vi "SPECAN_DPD_AMPM_ACP_TXP.vi"() -> ()   [LabVIEW 2016]
doc: "This example illustrates how to use the RFmx SpecAn and LTE personalities together with the RFSG drivers to perform ACP and EVM measurements with or without digital predistortion (DPD) of the waveform input to the DUT. \n\nDPD is a technique to optimize the operating point of power amplifiers and other non-linear RFIC devices. Power amplifiers are much more efficient if they operate near compression. However, compressing signal amplitudes can significantly deteriorate the amplified signal's quality both, in-band (e.g., EVM increases due to non-linear distortion of the signal's I/Q constellation) and out-of-band (e.g., ACP or SEM test fails due to spectral regrowth). With DPD, the original waveform is first pre-distorted in a way that matches the non-linear effects of the RFIC device before being fed through the device. The resulting output is a much cleaner amplified and/or filtered version of the original waveform. \n\nDifferent DPD models can be used to trade off performance with computational ease, with the Lookup-Table (LUT) model the simplest and the Generalized Memory Polynomial Model (GMP) the most complex. With a LUT, the DPD algorithm achieves gain and phase linearization on average. If you want to correct for memory effects - i.e., an output sample not only depends on the current input but also previous input samples; you will notice that a specific input power value translates into a range of gain and phase values - you would use one of the memory polynomial models. For these models, several parameters such as polynomial order and memory depth are available to fine-tune the model to the DUT behavior."
uses:
  <instrlib>/niRFSG/niRFSG.llb/niRFSG Exported Signal Destinations.ctl
  Source/SG/Typedefs/Instrument Configuration.ctl
  <instrlib>/niRFSG/niRFSG.llb/niRFSG Ref Clock Sources.ctl
  Source/Common/Local Oscillator Sharing Mode.ctl
  Source/SA/RFmxSpecAn/Typedefs/SpecAn AMPM Configuration.ctl
  Source/Common/Waveform.ctl
  Source/SA/RFmxSpecAn/Typedefs/SpecAn AMPM Results.ctl
  Source/Common/SA Common Configuration.ctl
  Source/SA/RFmxSpecAn/Typedefs/SpecAn ACP Configuration.ctl
  Source/SA/RFmxSpecAn/Typedefs/SpecAn ACP Component Carrier Configuration.ctl
  Source/SA/RFmxSpecAn/Typedefs/SpecAn ACP Offset Channel Configuration.ctl
  Source/SA/RFmxSpecAn/Typedefs/SpecAn ACP Offset Results.ctl
  Source/SA/RFmxSpecAn/Typedefs/SpecAn ACP Component Carrier Results.ctl
  Source/SA/RFmxSpecAn/Typedefs/SpecAn TxP Configuration.ctl
  Source/SA/RFmxSpecAn/Typedefs/SpecAn TxP Results.ctl
  Source/Methods/RFmxDPD/Typedefs/Common Configuration.ctl
  Source/Methods/RFmxDPD/Typedefs/Memory Polynomial Configuration.ctl
  Source/SA/RFmxInstr/Typedefs/Instrument Configuration.ctl
  Source/Methods/RFmxDPD/Typedefs/Pre DPD Crest Factor Reduction Configuration.ctl
  Source/Methods/RFmxDPD/Typedefs/Pre DPD Crest Factor Reduction Carrier Channel.ctl
  Source/Methods/RFmxDPD/Typedefs/Apply DPD Crest Factor Reduction Configuration.ctl
  Source/Common/SA Auto Level Configuration.ctl
  <vilib>/RFmx/SpecAn/mx/RFmxSpecAn.llb/RFmxSpecAn AMPM Fetch AM to AM Trace.vi
  <vilib>/RFmx/SpecAn/mx/RFmxSpecAn.llb/RFmxSpecAn AMPM Fetch AM to PM Trace.vi
  <vilib>/RFmx/SpecAn/mx/RFmxSpecAn.llb/RFmxSpecAn ACP Fetch Spectrum.vi
  <vilib>/RFmx/SpecAn/mx/RFmxSpecAn.llb/RFmxSpecAn TXP Fetch Power Trace.vi
  Source/SG/SG.lvlib
  Source/SA/RFmxSpecAn/RFmxSpecAn.lvlib
  Source/Methods/RFmxDPD/RFmxDPD.lvlib
  Source/SA/RFmxInstr/RFmxInstr.lvlib
  Source/Common/Common.lvlib
panel:
  in  "Display Tab Control":enum32{"AMPM Results", "ACP Results", "TxP"}(tab)
  out "AM to AM Plot":T1(graph)
  out "AM to PM Plot":T2(graph)
  out "AMPM Measurement Results":T3 {"AM to PM Residual (deg)" format="%.2f"; "AM to AM Residual (dB)" format="%.2f"; "Mean RMS EVM (%)" format="%.2f"; "1 dB Compression Point (dBm)" format="%.2f"; "Mean Linear Gain (dB)" format="%.2f"}
  out "Spectrum":cluster{"x0":dbl, "dx":dbl, "y":sgl[]}(graph) caption="DUT Output Spectrum"
  out "Offset Results":T4[](array[typedef])
  out "Component Carrier Results":T5[](array[typedef])
  out "Total Carrier Power (dBm or dBm/Hz)":dbl
  out "Power Trace":cluster{"x0":dbl, "dx":dbl, "y":sgl[]}(graph)
  out "TxP Results":T6 {"Minimum Power (dBm)" format="%.2f"; "Maximum Power (dBm)" format="%.2f"; "Peak to Average Ratio (dB)" format="%.2f"; "Average Mean Power (dBm)" format="%.2f"}
  in  "Measurement Settings Tab Control":T7(tab)
  in  "TxP Config":T8={"Measurement Interval (s)"=0.001, "RBW (Hz)"=20000000.0, "RBW Filter Type"=5, "RRC Alpha"=0.0, "Averaging Enabled"=0, "Averaging Count"=10, "Averaging Type"=0} {"Averaging Type" items=["RMS", "Log", "Scalar", "Max", "Min"]; "Averaging Enabled" items=["False", "True"]; "RRC Alpha" format="%.3g"; "RBW Filter Type" items=["None"=5, "Gaussian"=1, "Flat"=2, "RRC"=6]; "RBW (Hz)" format="%.3p"; "Measurement Interval (s)" format="%.2p"}
  in  "RFmx SpecAn AMPM Configuration":T9={"Measurement Interval (s)"=0.0001, "DUT Average Input Power (dBm)"=-20.0, "Signal Type"=0, "Reference Waveform"={"Name"="Wfm", "Data"=refnum, "Signal Bandwidth (Hz)"=0.0, "PAPR (dB)"=0.0, "Burst Length (s)"=0.0, "Sample Rate"=0.0, "Burst Start Locations"=[], "Burst Stop Locations"=[], "Idle Duration Present?"=FALSE, "Runtime Scaling"=0.0, "Script"=""}} {"Reference Waveform"."Runtime Scaling" format="%#_6p"; "Reference Waveform"."Sample Rate" format="%#_6p"; "Reference Waveform"."Burst Length (s)" format="%#_6p"; "Reference Waveform"."PAPR (dB)" format="%.2f"; "Reference Waveform"."Signal Bandwidth (Hz)" format="%#_6p"; "Signal Type" items=["Modulated", "Tones"]; "DUT Average Input Power (dBm)" format="%.2f"; "Measurement Interval (s)" format="%.2p"}
  in  "Common Configuration":T11={"Measurement Interval (s)"=0.0001, "Signal Type"=0, "DUT Average Input Power (dBm)"=-15.0, "Synchronization Method"=1} {"Synchronization Method" items=["Direct"=1, "Alias Protected"=2]; "DUT Average Input Power (dBm)" format="%.2f"; "Signal Type" items=["Modulated", "Tones"]; "Measurement Interval (s)" format="%#.2p"}
  in  "Memory Polynomial Configuration":T12={"Correction Type"=0, "Number of Iterations"=1, " Order"=3, " Depth"=2, "Lead Order"=2, "Lag Order"=2, "Lead Memory Depth"=2, "Lag Memory Depth"=2, "Maximum Lead"=2, "Maximum Lag"=2} {"Order" min=1; "Correction Type" items=["Magnitude and Phase", "Magnitude Only", "Phase Only"]}
  in  "Enable DPD":bool=TRUE
  in  "Pre DPD Crest Factor Reduction":T13={"Enabled"=0, "Method"=0, "Max Iterations"=10, "Target PAPR (dB)"=8.0, "Shaping Factor"=5.0, "Shaping Threshold (dB)"=-5.0, "Window Type"=7, "Window Length"=10, "Filter Enabled"=0, "Carrier Channels"=[{"Offset (Hz)"=0.0, "Bandwidth (Hz)"=20000000.0}]} {"Carrier Channels"."Bandwidth (Hz)" format="%.2p"; "Carrier Channels"."Offset (Hz)" format="%.2p"; "Filter Enabled" items=["False", "True"]; "Window Type" items=["Flat Top"=1, "Hanning"=2, "Hamming"=3, "Gaussian"=4, "Blackman"=5, "Blackman-Harris"=6, "Kaiser-Bessel"=7]; "Method" items=["Clipping", "Peak Windowing", "Sigmoid"]; "Enabled" items=["False", "True"]}
  in  "Apply DPD Crest Factor Reduction":T15={"Enabled"=0, "Method"=0, "Max Iterations"=10, "Target PAPR Type"=0, "Target PAPR (dB)"=8.0, "Window Type"=7, "Window Length"=10, "Shaping Factor"=5.0, "Shaping Threshold (dB)"=-5.0} {"Target PAPR Type" items=["Input PAPR", "Custom"]; "Window Type" items=["Flat Top"=1, "Hanning"=2, "Hamming"=3, "Gaussian"=4, "Blackman"=5, "Blackman-Harris"=6, "Kaiser-Bessel"=7]; "Method" items=["Clipping", "Peak Windowing", "Sigmoid"]; "Enabled" items=["False", "True"]}
  in  "ACP Configuration":T16={"Power Units"=0, "Averaging Enabled"=0, "Averaging Count"=10, "Averaging Type"=0, "FFT Window"=1, "FFT Padding"=-1.0, "RBW Auto"=1, "RBW (Hz)"=10000.0, "RBW Filter Type"=1, "Sweep Time Auto"=1, "Sweep Time Interval (s)"=0.001, "Component Carrier Configuration"=[], "Offset Channel Configuration"=[]} {"Offset Channel Configuration"."RRC Alpha" format="%.3g"; "Offset Channel Configuration"."RRC Filter Enabled" items=["False", "True"]; "Offset Channel Configuration"."Relative Attenuation (dB)" format="%.2f"; "Offset Channel Configuration"."Power Reference Carrier" items=["Closest", "Highest", "Composite", "Specific"]; "Offset Channel Configuration"."Sideband" items=["Neg", "Pos", "Both"]; "Offset Channel Configuration"."Frequency (Hz)" format="%.3p"; "Offset Channel Configuration"."Enabled" items=["False", "True"]; "Offset Channel Configuration"."Integration Bandwidth (Hz)" format="%.3p"; "Component Carrier Configuration"."RRC Alpha" format="%.3g"; "Component Carrier Configuration"."RRC Filter Enabled" items=["False", "True"]; "Component Carrier Configuration"."Mode" items=["Passive", "Active"]; "Component Carrier Configuration"."Frequency (Hz)" format="%.3p"; "Component Carrier Configuration"."Integration Bandwidth (Hz)" format="%.3p"; "Sweep Time Interval (s)" format="%.2p"; "Sweep Time Auto" items=["False", "True"]; "RBW Filter Type" items=["FFT Based", "Gaussian", "Flat", "Synch Tuned - 4", "Synch Tuned - 5"]; "RBW (Hz)" format="%.3p"; "RBW Auto" items=["False", "True"]; "FFT Padding" format="%.2f"; "FFT Window" items=["None", "Flat Top", "Hanning", "Hamming", "Gaussian", "Blackman", "Blackman-Harris", "Kaiser-Bessel"]; "Averaging Type" items=["RMS", "Log", "Scalar", "Max", "Min", "Vector"]; "Averaging Enabled" items=["False", "True"]; "Power Units" items=["dBm", "dBm/Hz"]}
  in  "Offset Channel Configuration":T18[](array[typedef])=[{"Integration Bandwidth (Hz)"=18000000.0, "Enabled"=1, "Frequency (Hz)"=20000000.0, "Sideband"=2, "Power Reference Carrier"=0, "Power Reference Specific Index"=0, "Relative Attenuation (dB)"=0.0, "RRC Filter Enabled"=0, "RRC Alpha"=0.22}, {"Integration Bandwidth (Hz)"=3840000.0, "Enabled"=1, "Frequency (Hz)"=12500000.0, "Sideband"=2, "Power Reference Carrier"=0, "Power Reference Specific Index"=0, "Relative Attenuation (dB)"=0.0, "RRC Filter Enabled"=0, "RRC Alpha"=0.22}, {"Integration Bandwidth (Hz)"=3840000.0, "Enabled"=1, "Frequency (Hz)"=17500000.0, "Sideband"=2, "Power Reference Carrier"=0, "Power Reference Specific Index"=0, "Relative Attenuation (dB)"=0.0, "RRC Filter Enabled"=0, "RRC Alpha"=0.22}] {"RRC Alpha" format="%.3g"; "RRC Filter Enabled" items=["False", "True"]; "Relative Attenuation (dB)" format="%.2f"; "Power Reference Carrier" items=["Closest", "Highest", "Composite", "Specific"]; "Sideband" items=["Neg", "Pos", "Both"]; "Frequency (Hz)" format="%.3p"; "Enabled" items=["False", "True"]; "Integration Bandwidth (Hz)" format="%.3p"}
  in  "Carrier Channel Configuration":T17[](array[typedef])=[{"Frequency (Hz)"=0.0, "Integration Bandwidth (Hz)"=18000000.0, "Mode"=1, "RRC Filter Enabled"=0, "RRC Alpha"=0.22}] {"RRC Alpha" format="%.3g"; "RRC Filter Enabled" items=["False", "True"]; "Mode" items=["Passive", "Active"]; "Frequency (Hz)" format="%.3p"; "Integration Bandwidth (Hz)" format="%.3p"}
  in  "Resource Control":enum32{"RFSG", "RFSA"}(tab)
  in  "Marker Event Output Terminal":T19="PXI_Trig0"
  in  "Reference Waveform File Path":path=path "C:/Users/Public/Documents/National Instruments/RFIC Test Software/Waveforms/LTE_FDD_UL_1x20MHz_256QAM_OS4.tdms"
  in  "RFSG Resource Name":refnum<k15>="RFSG"
  in  "SG Configuration":T20={"SelectedPorts"="", "Reference Clock Source"="PXI_CLK", "Carrier Frequency (Hz)"=3500000000.0, "DUT Average Input Power (dBm)"=-10.0, "External Attenuation (dB)"=0.0, "LO Sharing Mode"=enum."Automatic"}
  in  "RFSA Resource Name":refnum<k15>="RFSA"
  in  "RFmx SpecAn Configuration":T23={"Center Frequency (Hz)"=1000000000.0, "Reference Level (dBm)"=0.0, "External Attenuation (dB)"=0.0, "Trigger Enabled"=TRUE, "Digital Trigger Source"="PXI_Trig0", "Trigger Delay (s)"=0.0, "Selected Ports"=""} {"Trigger Delay (s)" format="%.2p"; "External Attenuation (dB)" format="%.2f"; "Reference Level (dBm)" format="%.2f"; "Center Frequency (Hz)" format="%.6p"}
  in  "Instrument Configuration":T24={"LO Sharing Mode"=enum."Automatic", "Frequency Reference Source"="PXI_Clk"}
  in  "Auto Level Configuration":T25={"Enabled"=TRUE, "Measurement Interval (s)"=0.01} {"Measurement Interval (s)" min=1e-06 max=100.0 format="%.2p"}
  in  "Auto Level Bandwidth (Hz)":dbl=20000000.0 format="%#_13p"
  in  "Center Frequency / SG IF (Hz)":dbl=3500000000.0 format="%.6p"
  in  "Error Tab Control":enum32{"Page 1", "Page 2"}(tab)
  out "error out":errorcluster
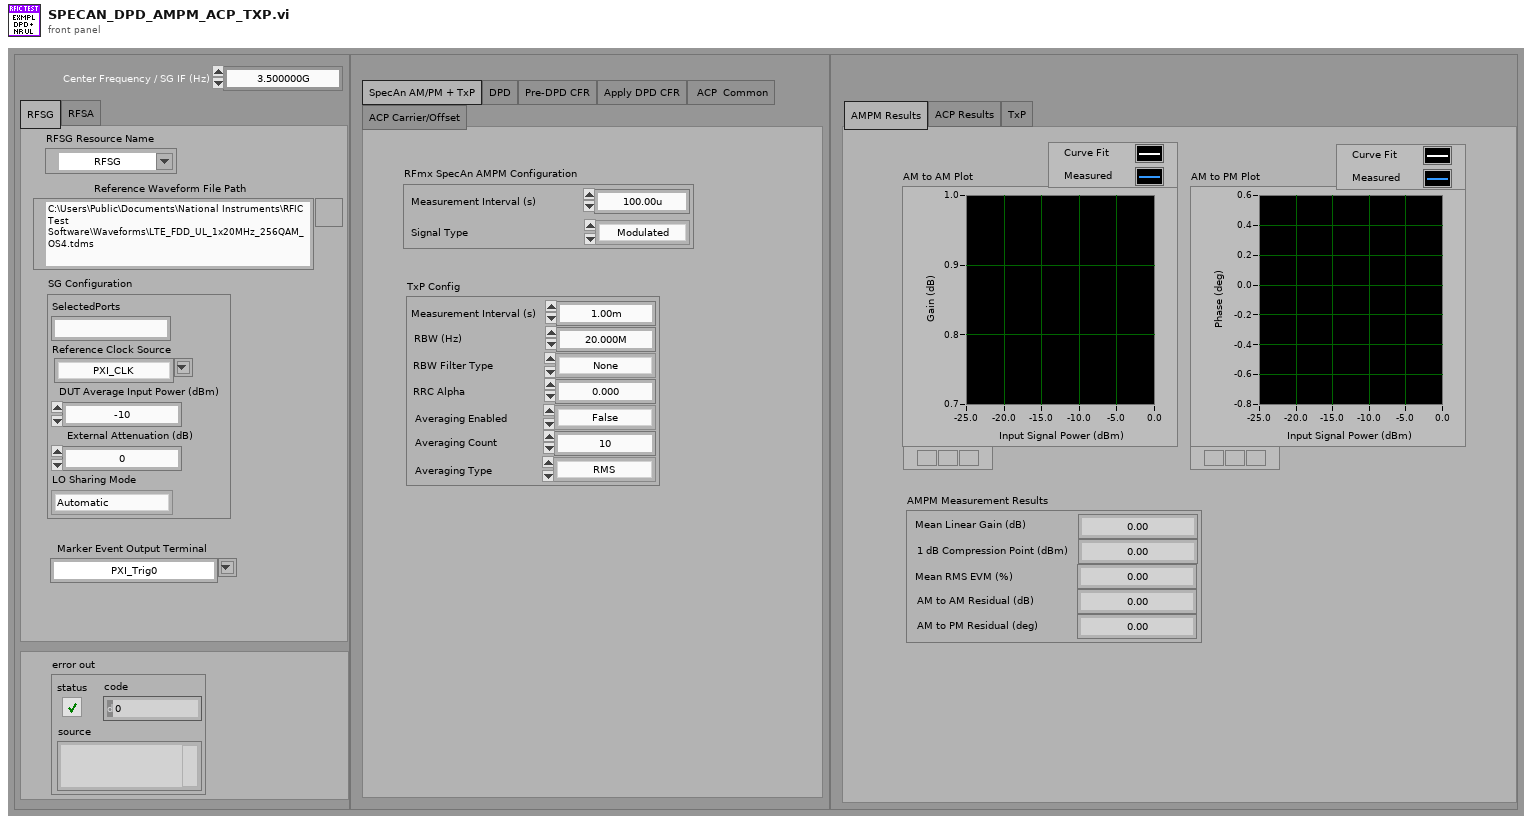
[diagram p1: front panel]
types:
  T1 = cluster{"Input Powers (dBm)":sgl[], "Curve Fit AM to AM (dB)":sgl[]}[]
  T2 = cluster{"Input Powers (dBm)":sgl[], "Curve Fit AM to PM (dB)":sgl[]}[]
  T3 = typedef "RFmxSpecAn.lvlib/SpecAn AMPM Results.ctl" = cluster{"Mean Linear Gain (dB)":dbl, "1 dB Compression Point (dBm)":dbl, "Mean RMS EVM (%)":dbl, "AM to AM Residual (dB)":dbl, "AM to PM Residual (deg)":dbl}
  T4 = typedef "RFmxSpecAn.lvlib/SpecAn ACP Offset Results.ctl" = cluster{"Lower Absolute Power (dBm)":dbl, "Upper Absolute Power (dBm)":dbl, "Lower Relative Power (dB)":dbl, "Upper Relative Power (dB)":dbl, "Frequency (Hz)":dbl, "Integration Bandwidth (Hz)":dbl}
  T5 = typedef "RFmxSpecAn.lvlib/SpecAn ACP Component Carrier Results.ctl" = cluster{"Frequency (Hz)":dbl, "Integration Bandwidth (Hz)":dbl, "Absolute Power (dBm or dBmHz)":dbl, "Total Relative Power (dB)":dbl}
  T6 = typedef "RFmxSpecAn.lvlib/SpecAn TxP Results.ctl" = cluster{"Average Mean Power (dBm)":dbl, "Peak to Average Ratio (dB)":dbl, "Maximum Power (dBm)":dbl, "Minimum Power (dBm)":dbl}
  T7 = enum32{"SpecAn AM/PM + TxP", "DPD", "Pre-DPD CFR", "Apply DPD CFR", " ACP  Common", "ACP Carrier/Offset"}
  T8 = typedef "RFmxSpecAn.lvlib/SpecAn TxP Configuration.ctl" = cluster{"Measurement Interval (s)":dbl, "RBW (Hz)":dbl, "RBW Filter Type":i32, "RRC Alpha":dbl, "Averaging Enabled":i32, "Averaging Count":i32, "Averaging Type":i32}
  T9 = typedef "RFmxSpecAn.lvlib/SpecAn AMPM Configuration.ctl" = cluster{"Measurement Interval (s)":dbl, "DUT Average Input Power (dBm)":dbl, "Signal Type":i32, "Reference Waveform":T10}
  T10 = typedef "Common.lvlib/Waveform.ctl" = cluster{"Name":string, "Data":refnum<data-value>, "Signal Bandwidth (Hz)":dbl, "PAPR (dB)":dbl, "Burst Length (s)":dbl, "Sample Rate":dbl, "Burst Start Locations":i32[], "Burst Stop Locations":i32[], "Idle Duration Present?":bool, "Runtime Scaling":dbl, "Script":string}
  T11 = typedef "RFmxDPD.lvlib/Common Configuration.ctl" = cluster{"Measurement Interval (s)":dbl, "Signal Type":i32, "DUT Average Input Power (dBm)":dbl, "Synchronization Method":i32}
  T12 = typedef "RFmxDPD.lvlib/Memory Polynomial Configuration.ctl" = cluster{"Correction Type":i32, "Number of Iterations":i32, " Order":i32, " Depth":i32, "Lead Order":i32, "Lag Order":i32, "Lead Memory Depth":i32, "Lag Memory Depth":i32, "Maximum Lead":i32, "Maximum Lag":i32}
  T13 = typedef "RFmxDPD.lvlib/Pre DPD Crest Factor Reduction Configuration.ctl" = cluster{"Enabled":i32, "Method":i32, "Max Iterations":i32, "Target PAPR (dB)":dbl, "Shaping Factor":dbl, "Shaping Threshold (dB)":dbl, "Window Type":i32, "Window Length":i32, "Filter Enabled":i32, "Carrier Channels":T14[]}
  T14 = typedef "RFmxDPD.lvlib/Pre DPD Crest Factor Reduction Carrier Channel.ctl" = cluster{"Offset (Hz)":dbl, "Bandwidth (Hz)":dbl}
  T15 = typedef "RFmxDPD.lvlib/Apply DPD Crest Factor Reduction Configuration.ctl" = cluster{"Enabled":i32, "Method":i32, "Max Iterations":i32, "Target PAPR Type":i32, "Target PAPR (dB)":dbl, "Window Type":i32, "Window Length":i32, "Shaping Factor":dbl, "Shaping Threshold (dB)":dbl}
  T16 = typedef "RFmxSpecAn.lvlib/SpecAn ACP Configuration.ctl" = cluster{"Power Units":i32, "Averaging Enabled":i32, "Averaging Count":i32, "Averaging Type":i32, "FFT Window":i32, "FFT Padding":dbl, "RBW Auto":i32, "RBW (Hz)":dbl, "RBW Filter Type":i32, "Sweep Time Auto":i32, "Sweep Time Interval (s)":dbl, "Component Carrier Configuration":T17[], "Offset Channel Configuration":T18[]}
  T17 = typedef "RFmxSpecAn.lvlib/SpecAn ACP Component Carrier Configuration.ctl" = cluster{"Frequency (Hz)":dbl, "Integration Bandwidth (Hz)":dbl, "Mode":i32, "RRC Filter Enabled":i32, "RRC Alpha":dbl}
  T18 = typedef "RFmxSpecAn.lvlib/SpecAn ACP Offset Channel Configuration.ctl" = cluster{"Integration Bandwidth (Hz)":dbl, "Enabled":i32, "Frequency (Hz)":dbl, "Sideband":i32, "Power Reference Carrier":i32, "Power Reference Specific Index":i32, "Relative Attenuation (dB)":dbl, "RRC Filter Enabled":i32, "RRC Alpha":dbl}
  T19 = typedef "niRFSG Exported Signal Destinations.ctl" = string
  T20 = typedef "SG.lvlib/Instrument Configuration.ctl" = cluster{"SelectedPorts":string, "Reference Clock Source":T21, "Carrier Frequency (Hz)":dbl, "DUT Average Input Power (dBm)":dbl, "External Attenuation (dB)":dbl, "LO Sharing Mode":T22}
  T21 = typedef "niRFSG Ref Clock Sources.ctl" = string
  T22 = typedef "Common.lvlib/Local Oscillator Sharing Mode.ctl" = enum16{"Automatic", "None"}
  T23 = typedef "Common.lvlib/SA Common Configuration.ctl" = cluster{"Center Frequency (Hz)":dbl, "Reference Level (dBm)":dbl, "External Attenuation (dB)":dbl, "Trigger Enabled":bool, "Digital Trigger Source":string, "Trigger Delay (s)":dbl, "Selected Ports":string}
  T24 = typedef "RFmxInstr.lvlib/Instrument Configuration.ctl" = cluster{"LO Sharing Mode":T22, "Frequency Reference Source":string}
  T25 = typedef "Common.lvlib/SA Auto Level Configuration.ctl" = cluster{"Enabled":bool, "Measurement Interval (s)":dbl}
  T26 = enum16{"ACP", "CCDF", "CHP", "FCnt", "Harmonics", "OBW", "SEM", "Spectrum", "Spur", "TXP", "AMPM", "DPD", "IQ", "IM", "NF", "PhaseNoise", "PAVT"}[]
  T27 = cluster{"Reference Powers (dBm)":sgl[], "Curve Fit AM to AM (dB)":sgl[]}
  T28 = cluster{"Reference Powers (dBm)":sgl[], "Measured AM to AM (dB)":sgl[]}
  T29 = cluster{"Reference Powers (dBm)":sgl[], "Curve Fit AM to PM (deg)":sgl[]}
  T30 = cluster{"Reference Powers (dBm)":sgl[], "Measured AM to PM (deg)":sgl[]}
  T31 = cluster{"Reference Powers (dBm)":sgl[], "Measured AM to AM (dB)":sgl[]}[]
  T32 = cluster{"Reference Powers (dBm)":sgl[], "Measured AM to PM (deg)":sgl[]}[]
  T33 = typedef "RFmxSpecAn.lvlib/SpecAn ACP Results.ctl" = cluster{"Total Carrier Power (dBm or dBm/Hz)":dbl, "Offset Results":T4[], "Component Carrier Results":T5[]}
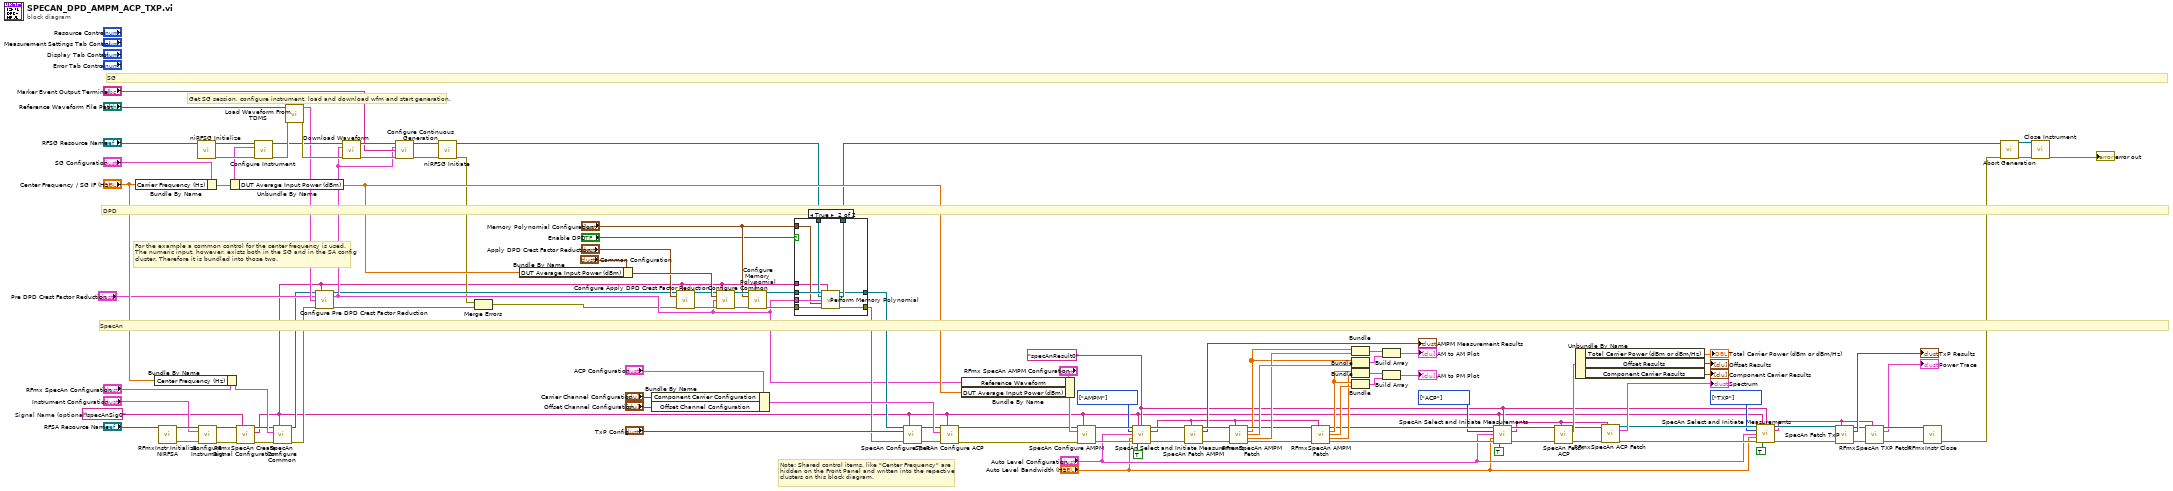
[diagram p0: block diagram]
diagram:
  w7 = "specAnResult0" ("Result Name")
  w4 = "specAnSig0"  # Signal Name (optional)
  w21 = T26 [enum."TXP"] items=["ACP", "CCDF", "CHP", "FCnt", "Harmonics", "OBW", "SEM", "Spectrum", "Spur", "TXP", "AMPM", "DPD", "IQ", "IM", "NF", "PhaseNoise", "PAVT"] ("Measurements")
  w27 = T26 [enum."ACP"] items=["ACP", "CCDF", "CHP", "FCnt", "Harmonics", "OBW", "SEM", "Spectrum", "Spur", "TXP", "AMPM", "DPD", "IQ", "IM", "NF", "PhaseNoise", "PAVT"] ("Measurements")
  w36 = T26 [enum."AMPM"] items=["ACP", "CCDF", "CHP", "FCnt", "Harmonics", "OBW", "SEM", "Spectrum", "Spur", "TXP", "AMPM", "DPD", "IQ", "IM", "NF", "PhaseNoise", "PAVT"] ("Measurements")
  # "DPD"
  # "Get SG session, configure instrument, load and download wfm and start generation."
  # "For the example a common control for the center frequency is used. \nThe numeric input, however, exists both in the SG and in the SA config\ncluster. Therefore it is bundled into those two."
  # "SpecAn"
  # "Note: Shared control items, like \"Center Frequency\" are \nhidden on the Front Panel and written into the repective \nclusters on this block diagram."
  # "SG"
  n1 = Bundle By Name(cluster="SG Configuration", "Carrier Frequency (Hz)"="Center Frequency / SG IF (Hz)") -> (w102:T20)
  n2 = Bundle By Name(cluster="RFmx SpecAn Configuration", "Center Frequency (Hz)"="Center Frequency / SG IF (Hz)") -> (w94:T23)
  n3 = call <vilib>:"RFmxInstr Initialize NIRFSA.vi"("Resource Name"="RFSA Resource Name") -> ("Instrument Handle Out"=w45:refnum<k21>, "error out"=w44:errorcluster)  [unwired: 12 in, 1 out]
  n4 = call <instrlib>:"niRFSG Initialize.vi"("resource name"="RFSG Resource Name") -> ("instrument handle"=w115:refnum<k15>, "error out"=w114:errorcluster)  [unwired: 13 in]
  n5 = call "Configure Instrument.vi"("Instrument Handle In"=w45, "Instrument Configuration"="Instrument Configuration", "error in (no error)"=w44) -> ("Instrument Handle Out"=w6:refnum<k21>, "error out"=w2:errorcluster)  [unwired: 11 in]
  n6 = Unbundle By Name(w102) -> ("DUT Average Input Power (dBm)"=w58:dbl)
  n7 = call <vilib>:"RFmxSpecAn Create Signal Configuration.vi"("Instrument Handle In"=w6, "Signal Name"=w4, "error in (no error)"=w2) -> ("Instrument Handle Out"=w5:refnum<k21>, "Selector String Out"=w3:string, "error out"=w1:errorcluster)  [unwired: 10 in]
  n8 = call "Configure Instrument.vi"("RFSG Session In"=w115, "SG Configuration"=w102, "error in (no error)"=w114) -> ("RFSG Session Out"=w119:refnum<k15>, "error out"=w121:errorcluster)  [unwired: 11 in]
  n9 = call "SpecAn Configure Common.vi"("RFmx Handle In"=w5, "Selector String"=w3, "Common Configuration"=w94, "error in (no error)"=w1) -> ("RFmx Handle Out"=w15:refnum<k21>, "error out"=w16:errorcluster)  [unwired: 10 in]
  n10 = call "Load Waveform From TDMS.vi"("TDMS File Path"="Reference Waveform File Path", "error in (no error)"=w121) -> ("Waveform"=w42:T10, "error out"=w120:errorcluster)  [unwired: 12 in]
  n11 = call "Configure Pre DPD Crest Factor Reduction.vi"("Instrument Handle In"=w15, "Selector String"=w3, "Pre DPD Crest Factor Reduction Configuration"="Pre DPD Crest Factor Reduction", "Reference Waveform"=w42, "error in (no error)"=w16) -> ("Instrument Handle Out"=w14:refnum<k21>, "Pre DPD CFR Waveform"=w17:T10, "error out"=w13:errorcluster)  [unwired: 8 in]
  n12 = call "Download Waveform.vi"("RFSG handle"=w119, "Waveform In"=w17, "error in (no error)"=w120) -> ("RFSG handle out"=w113:refnum<k15>, "error out"=w111:errorcluster)  [unwired: 11 in]
  n13 = call "Configure Continuous Generation.vi"("RFSG handle"=w113, "Waveform in"=w17, "Waveform Start Trigger Export"="Marker Event Output Terminal", "error in"=w111) -> ("RFSG handle out"=w112:refnum<k15>, "error out"=w50:errorcluster)  [unwired: 9 in, 1 out]
  n14 = call <instrlib>:"niRFSG Initiate.vi"("instrument handle"=w112, "error in"=w50) -> ("instrument handle out"=w55:refnum<k15>, "error out"=w11:errorcluster)  [unwired: 12 in]
  n15 = Merge Errors(w11, w13) -> (w12:errorcluster)
  n16 = Bundle By Name(cluster="Common Configuration", "DUT Average Input Power (dBm)"=w58) -> (w59:T11)
  n17 = Bundle By Name(cluster="ACP Configuration", "Component Carrier Configuration"="Carrier Channel Configuration", "Offset Channel Configuration"="Offset Channel Configuration") -> (w89:T16)
  n18 = call "Configure Apply DPD Crest Factor Reduction.vi"("Instrument Handle In"=w14, "Selector String"=w3, "Apply DPD Crest Factor Reduction Configuration"="Apply DPD Crest Factor Reduction", "error in (no error)"=w12) -> ("Instrument Handle Out"=w40:refnum<k21>, "error out"=w39:errorcluster)  [unwired: 10 in]
  n19 = call "Configure Common.vi"("Instrument Handle In"=w40, "Selector String"=w3, "Common Configuration"=w59, "Reference Waveform"=w17, "error in (no error)"=w39) -> ("Instrument Handle Out"=w62:refnum<k21>, "error out"=w61:errorcluster)  [unwired: 9 in]
  n20 = call "Configure Memory Polynomial.vi"("Instrument Handle In"=w62, "Selector String"=w3, "Memory Polynomial Configuration"="Memory Polynomial Configuration", "error in (no error)"=w61) -> ("Instrument Handle Out"=w57:refnum<k21>, "error out"=w49:errorcluster)  [unwired: 10 in]
  n21 = case shown="True" "Enable DPD" {
    tunnel: w57 -> [w123 w133]
    tunnel: [w122 w132] -> w48
    tunnel: "Memory Polynomial Configuration" -> [_ w126]
    tunnel: w17 -> [_ w131]
    tunnel: w55 -> [w124 w130]
    tunnel: [w124 w129] -> w54
    tunnel: [w123 w128] -> w47
    tunnel: w49 -> [w122 w127]
    tunnel: w3 -> [_ w125]
    frame False {
    }
    frame True {
      n22 = call "Perform Memory Polynomial.vi"("RFmx Instrument Handle In"=w133, "Selector String"=w125, "RFSG Instrument Handle In"=w130, "Reference Waveform"=w131, "Memory Polynomial Configuration"=w126, "error in (no error)"=w127) -> ("RFmx Instrument Handle Out"=w128:refnum<k21>, "RFSG Instrument Handle Out"=w129:refnum<k15>, "error out"=w132:errorcluster)  [unwired: 6 in, 1 out]
    }
  }
  n23 = call "SpecAn Configure TxP.vi"("Instrument Handle In"=w47, "Selector String"=w3, "TxP Config"="TxP Config", "error in (no error)"=w48) -> ("Instrument Handle Out"=w51:refnum<k21>, "error out"=w92:errorcluster)  [unwired: 10 in]
  n24 = call "SpecAn Configure ACP.vi"("Instrument Handle In"=w51, "Selector String"=w3, "ACP Configuration"=w89, "error in (no error)"=w92) -> ("Instrument Handle Out"=w52:refnum<k21>, "error out"=w97:errorcluster)  [unwired: 10 in]
  n25 = Bundle By Name(cluster="RFmx SpecAn AMPM Configuration", "Reference Waveform"=w17, "DUT Average Input Power (dBm)"=w58) -> (w103:T9)
  n26 = call "SpecAn Configure AMPM.vi"("RFmx Handle In"=w52, "Selector String"=w3, "RFmx SpecAn AMPM Configuration"=w103, "error in (no error)"=w97) -> ("RFmx Handle Out"=w37:refnum<k21>, "error out"=w35:errorcluster)  [unwired: 10 in]
  n27 = call "SpecAn Select and Initiate Measurements.vi"("Instrument Handle In"=w37, "Selector String"=w3, "Result Name"=w7, "Measurements"=w36, "Auto Level Configuration"="Auto Level Configuration", "Auto Level Bandwidth (Hz)"="Auto Level Bandwidth (Hz)", "error in (no error)"=w35, "Enable All Traces (F)"=TRUE) -> ("Instrument Handle Out"=w33:refnum<k21>, "Selector String Out"=w10:string, "error out"=w34:errorcluster)  [unwired: 5 in]
  n28 = call "SpecAn Fetch AMPM.vi"("RFmx Handle In"=w33, "Selector String"=w10, "error in (no error)"=w34) -> ("RFmx Handle Out"=w80:refnum<k21>, "AMPM Results"=→"AMPM Measurement Results":T3, "error out"=w78:errorcluster)  [unwired: 10 in]
  n29 = call-poly <vilib>:"RFmxSpecAn AMPM Fetch.vi"("Instrument Handle In"=w80, "Selector String"=w10, "error in (no error)"=w78) -> ("Instrument Handle Out"=w79:refnum<k21>, "Reference Powers (dBm)"=w46:sgl[], "Measured AM to AM (dB)"=w85:sgl[], "Curve Fit AM to AM (dB)"=w84:sgl[], "error out"=w77:errorcluster)  [unwired: 8 in]
  n30 = call-poly <vilib>:"RFmxSpecAn AMPM Fetch.vi"("Instrument Handle In"=w79, "Selector String"=w10, "error in (no error)"=w77) -> ("Instrument Handle Out"=w31:refnum<k21>, "Reference Powers (dBm)"=w83:sgl[], "Measured AM to PM (deg)"=w82:sgl[], "Curve Fit AM to PM (deg)"=w81:sgl[], "error out"=w30:errorcluster)  [unwired: 8 in]
  n31 = Bundle("Reference Powers (dBm)"=w46, "Curve Fit AM to AM (dB)"=w84) -> (w76:T27)  [unwired: 1 in]
  n32 = Bundle("Reference Powers (dBm)"=w46, "Measured AM to AM (dB)"=w85) -> (w75:T28)  [unwired: 1 in]
  n33 = Bundle("Reference Powers (dBm)"=w83, "Curve Fit AM to PM (deg)"=w81) -> (w73:T29)  [unwired: 1 in]
  n34 = Bundle("Reference Powers (dBm)"=w83, "Measured AM to PM (deg)"=w82) -> (w74:T30)  [unwired: 1 in]
  n35 = Build Array(w76, w75) -> (→"AM to AM Plot":T31)
  n36 = Build Array(w73, w74) -> (→"AM to PM Plot":T32)
  n37 = call "SpecAn Select and Initiate Measurements.vi"("Instrument Handle In"=w31, "Selector String"=w3, "Result Name"=w7, "Measurements"=w27, "Auto Level Configuration"="Auto Level Configuration", "Auto Level Bandwidth (Hz)"="Auto Level Bandwidth (Hz)", "error in (no error)"=w30, "Enable All Traces (F)"=TRUE) -> ("Instrument Handle Out"=w29:refnum<k21>, "Selector String Out"=w9:string, "error out"=w28:errorcluster)  [unwired: 5 in]
  n38 = call "SpecAn Fetch ACP.vi"("RFmx Handle In"=w29, "Selector String"=w9, "error in (no error)"=w28) -> ("RFmx Handle Out"=w72:refnum<k21>, "ACP Results"=w96:T33, "error out"=w71:errorcluster)  [unwired: 10 in]
  n39 = Unbundle By Name(w96) -> ("Total Carrier Power (dBm or dBm/Hz)"=→"Total Carrier Power (dBm or dBm/Hz)":dbl, "Offset Results"=→"Offset Results":T4[], "Component Carrier Results"=→"Component Carrier Results":T5[])
  n40 = call-poly <vilib>:"RFmxSpecAn ACP Fetch.vi"("Instrument Handle In"=w72, "Selector String"=w9, "error in (no error)"=w71) -> ("Instrument Handle Out"=w25:refnum<k21>, "Spectrum (dBm or dBm/Hz)"=→"Spectrum":cluster{"x0":dbl, "dx":dbl, "y":sgl[]}, "error out"=w23:errorcluster)  [unwired: 10 in]
  n41 = call "SpecAn Select and Initiate Measurements.vi"("Instrument Handle In"=w25, "Selector String"=w3, "Result Name"=w7, "Measurements"=w21, "Auto Level Configuration"="Auto Level Configuration", "Auto Level Bandwidth (Hz)"="Auto Level Bandwidth (Hz)", "error in (no error)"=w23, "Enable All Traces (F)"=TRUE) -> ("Instrument Handle Out"=w24:refnum<k21>, "Selector String Out"=w8:string, "error out"=w22:errorcluster)  [unwired: 5 in]
  n42 = call "SpecAn Fetch TxP.vi"("Instrument Handle In"=w24, "Selector String"=w8, "error in (no error)"=w22) -> ("Instrument Handle Out"=w69:refnum<k21>, "TxP Results"=→"TxP Results":T6, "error out"=w67:errorcluster)  [unwired: 10 in]
  n43 = call-poly <vilib>:"RFmxSpecAn TXP Fetch.vi"("Instrument Handle In"=w69, "Selector String"=w8, "error in (no error)"=w67) -> ("Instrument Handle Out"=w68:refnum<k21>, "Power (dBm)"=→"Power Trace":cluster{"x0":dbl, "dx":dbl, "y":sgl[]}, "error out"=w66:errorcluster)  [unwired: 10 in]
  n44 = call <vilib>:"RFmxInstr Close.vi"("Instrument Handle In"=w68, "error in (no error)"=w66) -> ("error out"=w105:errorcluster)  [unwired: 13 in]
  n45 = call "Abort Generation.vi"("RFSG handle"=w54, "error in (no error)"=w105) -> ("RFSG handle out"=w118:refnum<k15>, "error out"=w117:errorcluster)  [unwired: 12 in]
  n46 = call "Close Instrument.vi"("RFSG Handle"=w118, "error in (no error)"=w117) -> ("error out"=→"error out":errorcluster)  [unwired: 13 in]
